vi "Read XML HW Configuration File_Extra Checks_Check Label Settings Uniqueness For Each hardWareChannel.vi"(8 "error in (no error)":errorcluster, 11 "Array In":T1[](array[typedef]) {"speed" items=["Auto", "Low", "High"]; "Labels"."scheduleBuildUnit" items=["Millisecond", "Microsecond"]}) -> (0 "error out":errorcluster)   [LabVIEW 2020]
doc: "This VI checks that for a given Hardware Channel, each Label Decimal and SDI settings is unique. If there are multiple duplicates, the function returns all duplicates."
uses:
  Controls/Ballard_Channel.ctl
  Controls/Ballard_Label.ctl
  Controls/Ballard_Word.ctl
  Controls/ARINCParam.ctl
  Shared/Controls and Global/TransferType.ctl
  Controls/Channel_direction.ctl
  Controls/Channel Speed.ctl
  <userlib>/_OpenG.lib/md5/md5.llb/MD5 Message Digest (Binary String)__ogtk.vi
  <userlib>/_OpenG.lib/array/array.llb/Remove Duplicates from 1D Array (String)__ogtk.vi
  Shared/Ballard Arinc-429 Shared.lvlib
  Ballard Arinc-429 System Explorer.lvlib
panel:
  out "Error Source":string
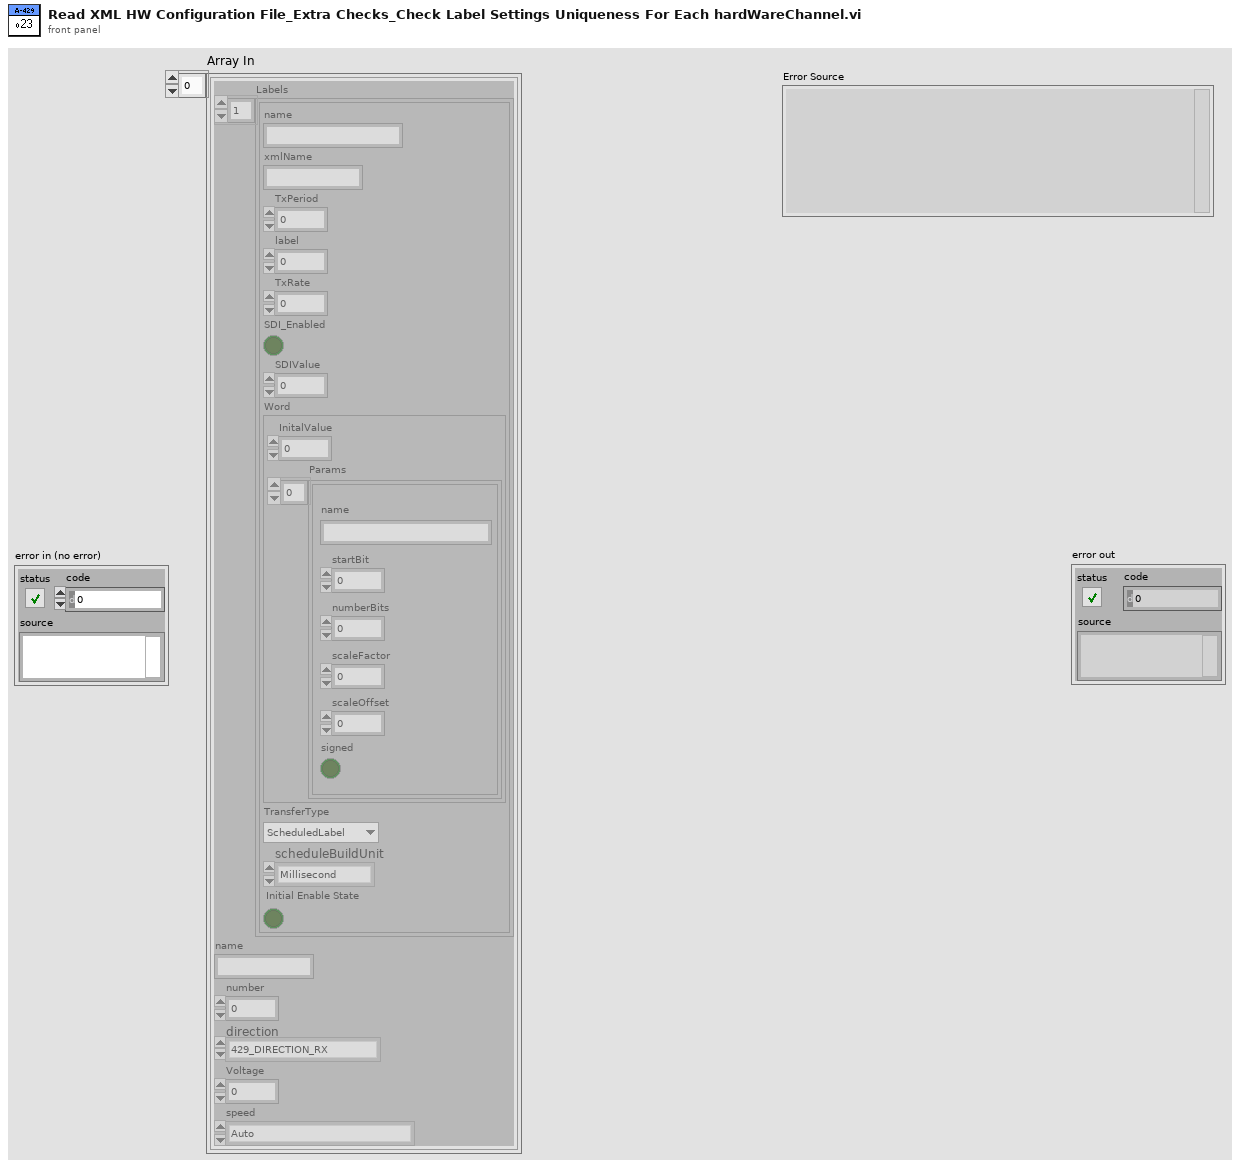
[diagram p1: front panel]
types:
  T1 = typedef "Ballard Arinc-429 System Explorer.lvlib/Ballard_Channel.ctl" = cluster{"Labels":T2[], "name":string, "number":u8, "direction":T6, "Voltage":dbl, "speed":T7}
  T2 = typedef "Ballard Arinc-429 System Explorer.lvlib/Ballard_Label.ctl" = cluster{"name":string, "xmlName":string, "TxPeriod":u32, "label":u32, "TxRate":dbl, "SDI_Enabled":bool, "SDIValue":u8, "Word":T3, "TransferType":T5, "scheduleBuildUnit":i32, "Initial Enable State":bool}
  T3 = typedef "Ballard Arinc-429 System Explorer.lvlib/Ballard_Word.ctl" = cluster{"InitalValue":u32, "Params":T4[]}
  T4 = typedef "Ballard Arinc-429 System Explorer.lvlib/ARINCParam.ctl" = cluster{"name":string, "startBit":i32, "numberBits":i32, "scaleFactor":dbl, "scaleOffset":dbl, "signed":bool}
  T5 = typedef "Ballard Arinc-429 Shared.lvlib/TransferType.ctl" = enum16{"ScheduledLabel", "Acyclic", "Block", "Strobe"}
  T6 = typedef "Ballard Arinc-429 System Explorer.lvlib/Channel_direction.ctl" = enum16{"429_DIRECTION_RX", "429_DIRECTION_TX"}
  T7 = typedef "Ballard Arinc-429 System Explorer.lvlib/Channel Speed.ctl" = i32
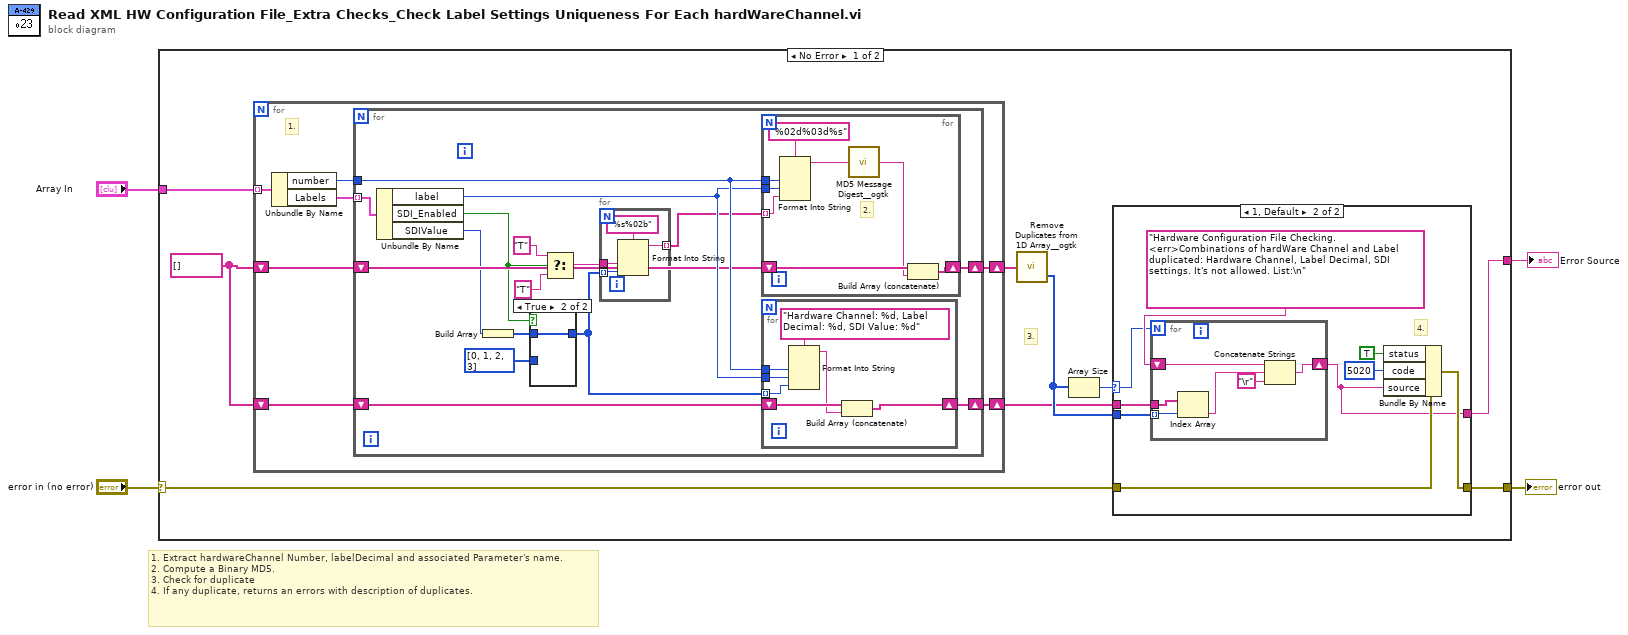
[diagram p0: block diagram]
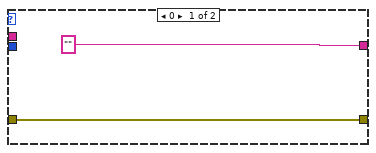
[diagram p2: hidden frame]
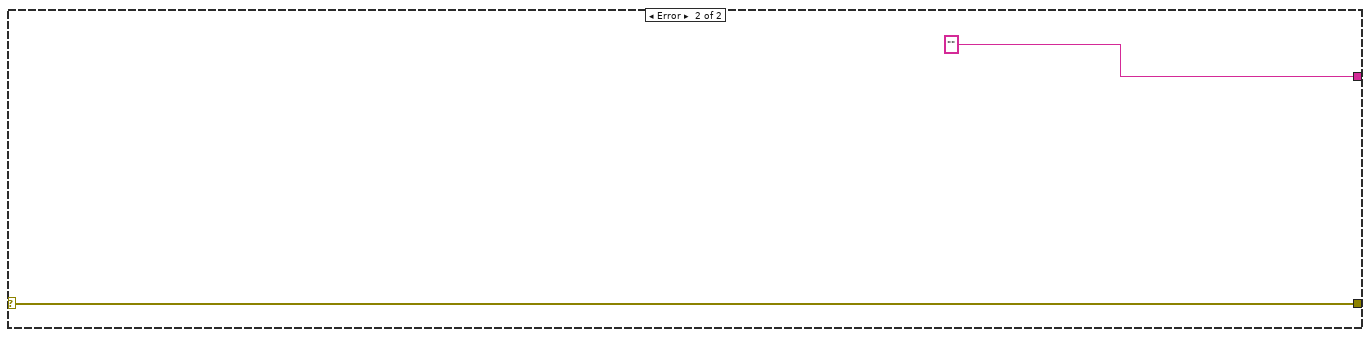
[diagram p4: hidden frame]
diagram:
  # "1. Extract hardwareChannel Number, labelDecimal and associated Parameter's name.\n2. Compute a Binary MD5.\n3. Check for duplicate\n4. If any duplicate, returns an errors with description of duplicates."
  n1 = case shown="No Error" "error in (no error)" {
    selector: "error in (no error)" -> [w12 w76]
    tunnel: [w9 w76] -> w3
    tunnel: "Array In" -> [w11 _]
    tunnel: [w8 ""] -> w1
    frame No Error {
      w6 = string[] []
      # "3."
      n2 = for {
        tunnel: w11 -> [w37] mode=indexing
        shift-right: [w33] -> w7
        shift-left: w6 -> [w34]
        shift-right: [w31] -> w5
        shift-left: w6 -> [w32]
        # "1."
        n3 = Unbundle By Name(w37) -> ("number"=w36:u8, "Labels"=w35:T2[])
        n4 = for {
          tunnel: w36 -> [w53]
          tunnel: w35 -> [w52] mode=indexing
          shift-right: [w49] -> w33
          shift-left: w34 -> [w50]
          shift-right: [w47] -> w31
          shift-left: w32 -> [w48]
          n5 = Unbundle By Name(w52) -> ("label"=w51:u32, "SDI_Enabled"=w46:bool, "SDIValue"=w45:u8)
          n6 = Build Array(w45) -> (w42:u8[])
          n7 = case shown="True" w46 {
            tunnel: w42 -> [_ w59]
            tunnel: i32[] [0, 1, 2, 3] -> [w58 _]
            tunnel: [w58 w59] -> w38
            frame False {
            }
            frame True {
            }
          }
          n8 = Select(t="T", s=w46, f="T") -> (s? t:f=w40:string)
          n9 = for {
            tunnel: w40 -> [w57]
            tunnel: w38 -> [w55] mode=indexing
            tunnel: [w54] -> w44 mode=indexing
            n10 = Format Into String(format string="%s%02b", w57, w55) -> (resulting string=w54:string)  [unwired: 2 in, 1 out]
          }
          n11 = for {
            tunnel: w53 -> [w74]
            tunnel: w51 -> [w73]
            tunnel: w44 -> [w67] mode=indexing
            shift-right: [w71] -> w49
            shift-left: w50 -> [w72]
            # "2."
            n12 = Format Into String(format string="%02d%03d%s", w74, w73, w67) -> (resulting string=w69:string)  [unwired: 2 in, 1 out]
            n13 = call-poly <userlib>:"MD5 Message Digest__ogtk.vi"("Message"=w69) -> ("MD5 Message Digest"=w68:string)
            n14 = Build Array (concatenate)(w72, w68) -> (w71:string[])
          }
          n15 = for {
            tunnel: w53 -> [w66]
            tunnel: w51 -> [w65]
            tunnel: w38 -> [w60] mode=indexing
            shift-right: [w63] -> w47
            shift-left: w48 -> [w64]
            n16 = Format Into String(format string="Hardware Channel: %d, Label Decimal: %d, SDI Value: %d", w66, w65, w60) -> (resulting string=w61:string)  [unwired: 2 in, 1 out]
            n17 = Build Array (concatenate)(w64, w61) -> (w63:string[])
          }
        }
      }
      n18 = call-poly <userlib>:"Remove Duplicates from 1D Array__ogtk.vi"("Input Array"=w7) -> ("indices of removed elements"=w10:i32[])  [unwired: 1 out]
      n19 = Array Size(array=w10) -> (size(s)=w13:i32)
      n20 = case shown="1, Default" w13 {
        selector: w13 -> [_ w19]
        tunnel: w12 -> [w15 w24]
        tunnel: w10 -> [_ w18]
        tunnel: [w15 w23] -> w9
        tunnel: ["" w17] -> w8
        tunnel: w5 -> [_ w16]
        frame 0 {
        }
        frame 1, Default {
          # "4."
          n21 = for {
            N: w19 -> [_]
            shift-right: [w29] -> w17
            shift-left: "Hardware Configuration File Checking.<err>Combinations of hardWare Channel and Label duplicated: Hardware Channel, Label Decimal, SDI settings. It's not allowed. List:\n" -> [w30]
            tunnel: w18 -> [w28] mode=indexing
            tunnel: w16 -> [w26]
            n22 = Index Array(array=w26, index=w28) -> (element=w25:string)
            n23 = Concatenate Strings(w30, w25, "\r") -> (w29:string)
          }
          n24 = Bundle By Name(cluster=w24, "status"=TRUE, "code"=5020, "source"=w17) -> (w23:errorcluster)
        }
      }
    }
    frame Error {
    }
  }
  "error out" <- w3
  "Error Source" <- w1
